vi "RHRT-IGVC-2013.vi"() -> ()   [LabVIEW 2011]
doc: "This the Rose-Hulman Robotics Tream IGVC compatition Code\nexample demonstrates the control of an autonomous robot through multiple asynchronous processes, modeled by VIs, that communicate with each other using shared variables. This example also shows an obstacle avoidance algorithm that the simulated robot uses as it navigates. The application includes the following processes:\n\n1. LIDAR Loop (\"Sense\")--Uses LabVIEW dataflow programming to generate simulated sensor data based on the position of the robot and any obstacles in the environment.\n\n2. Operator Loop (\"Think\")--Uses a state machine to control the movement of the robot according to commands from the user. When the robot follows a path without joystick or keyboard control, this process controls the attitude of the autonomous robot using a Vector Field Histogram (VFH) algorithm to avoid obstacles.\n\n3. Motor Loop (\"Act\")--Uses a Control and Simulation Loop, from the Control Design and Simulation Module, to create a model of the robot, simulate its dynamic behavior, and show the control loops and attitude observers."
uses:
  <vilib>/robotics/Controls/Compass Indicator/Compass Indicator.xctl
  <vilib>/Platform/TimedLoop/XDataNode/timing_clust.ctl
  <vilib>/Platform/TimedLoop/XDataNode/nitl_modes.ctl
  <vilib>/Platform/TimedLoop/XDataNode/wakeup.ctl
  <vilib>/Platform/TimedLoop/XDataNode/XDataNode.xnode
  <vilib>/Platform/TimedLoop/XDataNode/XDNodeRunTimeDep.lvlib
panel:
  out "Error":bool
  out "OK":bool
  in  "HUD 2":enum32{"GPS", "LIDAR", "IMU", "Occupancy Grid"}(tab)
  out "Health":u8(slide) scale=0.0..12.0
  out "XY Graph 2":cluster{dbl[], dbl[]}(graph)
  out "Data Aquired 2":picture
  out "Digree 2":dbl=16.3201904296875 caption="Digree"
  out "Compass Indicator 2":dbl(xcontrol)=16.3201904296875
  out "Occupancy Grid":dbl[][](graph)
  in  "Telemetry":T1(tab)
  out "Voltage":cluster{sgl, sgl, sgl}(knob)={13.4, 12.0, 47.48} caption="Main Battery Voltage\nInternal Voltage\nDSUB Voltage" scale=8.0..15.0
  out "Current":cluster{sgl, sgl, sgl, sgl}(knob)={0.0, 0.0, -2.0, -2.0} caption="Ch1 Motor Curret\nCh2 Motor Curret\nCh1 Battery Curret \nCh2 Battery Curret" scale=0.0..15.0
  out "IC Temp (C)":i32(slide)=22 scale=0.0..150.0
  out "Ch1 Temp (C)":i32(slide)=22 scale=0.0..150.0
  out "Ch2 Temp (C)":i32(slide)=23 scale=0.0..150.0
  out "Ch1 Encoder Speed\nCh2 Encoder Speed":cluster{i32, i32}(knob) scale=-300.0..300.0
  out "Image Out":T2(plugin-control)
  in  "Search For VISA":bool
  in  "HUD":T3(tab)=enum."Info"
  in  "Analog Stick":cluster{dbl, dbl}[](graph)
  in  "Clear Breadcrumbs":bool
  in  "Max Points":dbl=3000.0 format="%0.2f"
  out "XY Graph":cluster{dbl[], dbl[]}[](graph)
  out "Longitude Point":dbl format="%#_12g"
  out "Latitude Point":dbl format="%#_12g"
  out "Data Aquired":picture
  in  "Max Distance":dbl=3000.0 format="%0.2f"
  out "Digree":dbl=16.3201904296875
  out "Compass Indicator":dbl(xcontrol)=16.3201904296875
  out "Curretn POI":string
  in  "Curent Index":i32
  in  "Waypoint Table":string[][](table)=[["1.000000", "39.400000", "-87.200000"], ["2.000000", "39.600000", "-87.300000"], ["2.000000", "39.200000", "-87.400000"]]
  in  "Show GPS Diagram":bool
  in  "Show LL Diagram":bool
  in  "Show AI Diagram":bool
  in  "Show MCL Diagram":bool
  in  "About":bool
  in  "Stop":bool
  in  "Error Display":T4(tab)
  out "Cammera Status":bool
  out "Cammera Status 2":bool
  out "IMU Status":bool
  in  "IMU VISA":refnum<visa-resource-name>="COM7"
  out "Motor Status":bool
  in  "Motor VISA":refnum<visa-resource-name>="COM21"
  out "LIDAR Status":bool
  in  "LIDAR VISA":refnum<visa-resource-name>="COM20"
  out "GPS Status":bool
  in  "GPS VISA":refnum<visa-resource-name>="COM22"
  in  "GPS Error":errorcluster
  in  "LIDAR Error":errorcluster
  in  "Motor Error":errorcluster
  in  "IMU Error":errorcluster
  in  "Camera Error":errorcluster
  in  "Robot Mode:":T5(ring)
  out "End Loop":bool=TRUE
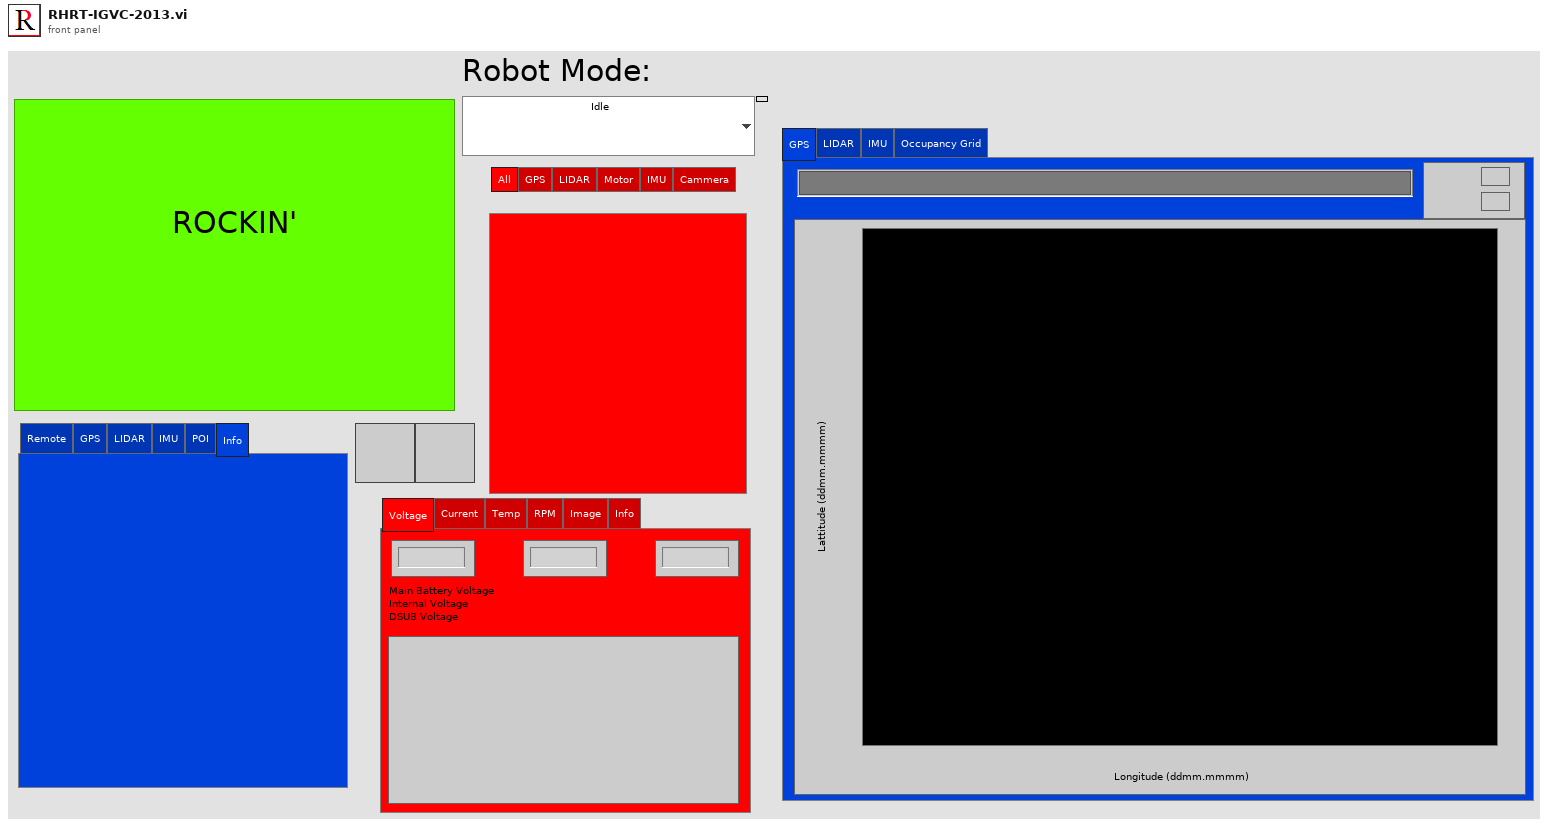
[diagram p1: front panel]
types:
  T1 = enum32{"Voltage", "Current", "Temp", "RPM", "Image", "Info"}
  T2 = typedef "IMAQ Image.ctl" = refnum<image>
  T3 = enum32{"Remote", "GPS", "LIDAR", "IMU", "POI", "Info"}
  T4 = enum32{"All", "GPS", "LIDAR", "Motor", "IMU", "Cammera"}
  T5 = enum16{"Idle", "Wiimote", "Joypad", "IGVC", "Avoide Objects", "Avoide Lines", "Path Planning", "Heading", "Waypoint"}
  T6 = typedef "XDNodeRunTimeDep.lvlib/timing_clust.ctl" = cluster{"Expected End [f-1]":u64, "Actual End [f-1]":u64, "Finished Late? [f-1]":bool, "Expected End [i-1]":u64, "Actual End [i-1]":u64, "Finished Late? [i-1]":bool, "Expected Start [i]":u64, "Actual Start [i]":u64, "Expected Start [f]":u64, "Actual Start [f]":u64, "Source Name":string, "Structure Name":string, "Period":i64, "Deadline":i64, "Offset":i64, "Start":i64, "Priority":i32, "Timeout":i32, "Mode":T7, "Wakeup Reason":T8, "Error":errorcluster, "Source Type":string, "Secondary Source Type":string, "Global End Time":u64, "Global Start Time":u64, "Frame Duration":u64, "Iteration Duration":u64, "Assigned CPU":i32, "I/O Scan Engine Mode":u32}
  T7 = typedef "XDNodeRunTimeDep.lvlib/nitl_modes.ctl" = enum32{"No Change", "Process missed periods, maintain original phase", "Discard missed periods, maintain original phase", "Process missed periods, ignore original phase", "Discard missed periods, ignore original phase"}
  T8 = typedef "XDNodeRunTimeDep.lvlib/wakeup.ctl" = enum32{"Normal", "Aborted", "Asynchronous wakeup", "Timing source error", "Timed loop error", "Timeout"}
  T9 = cluster{"Latitude":dbl, "Longitude":dbl, "Altitude":dbl, "Velocity, Correction & SET":cluster{"Velocity North":dbl, "Velocity East":dbl, "Velocity Up":dbl, "Ellipsoidal Height":dbl, "GDOP":sgl, "PDOP":sgl, "HDOP":sgl, "VDOP":sgl, "TDOP":sgl, "Horizontal Figure of Merit":u8, "Time Figure of Merit":u8, "Max dGPS Age":sgl, "Extended Navigation Mode":u8, "Antenna Height Adjustment ":dbl, "SET North":i32, "SET East":i32, "SET Up":i32}, "Time":cluster{"GPS Week":u16, "GPS Time of Week":sgl}, "Satellites Used":i32[]}
  T10 = cluster{"Azimuth":dbl, "FocusPointAltitude":dbl, "altMode":i32, "FocusPointLatitude":dbl, "FocusPointLongitude":dbl, "Range":dbl, "Tilt":dbl}
  T11 = cluster{"Position":cluster{"Roll":dbl, "Pitch":dbl, "Yaw":dbl}, "Orientation Matrix":dbl[][], "Magnetic Field":cluster{"Z-Axis Magnetic Field":dbl, "Y-Axis Magnetic Field":dbl, "X-Axis Magnetic Field":dbl}, "Acceleration":cluster{"Z-Axis Acceleration":dbl, "Y-Axis Acceleration":dbl, "X-Axis Acceleration":dbl}, "Angular Rate":cluster{"X-Axis Angular Rate":dbl, "Y-Axis Angular Rate":dbl, "Z-Axis Angular Rate":dbl}, "Quaternion":dbl[]}
  T12 = cluster{"Voltage":cluster{sgl, sgl, sgl}, "Encoder Speed":cluster{i32, i32}, "Temps":cluster{"IC Temp (C)":i32, "Ch1 Temp (C)":i32, "Ch2 Temp (C)":i32}, "Current":cluster{dbl, dbl, dbl, dbl}}
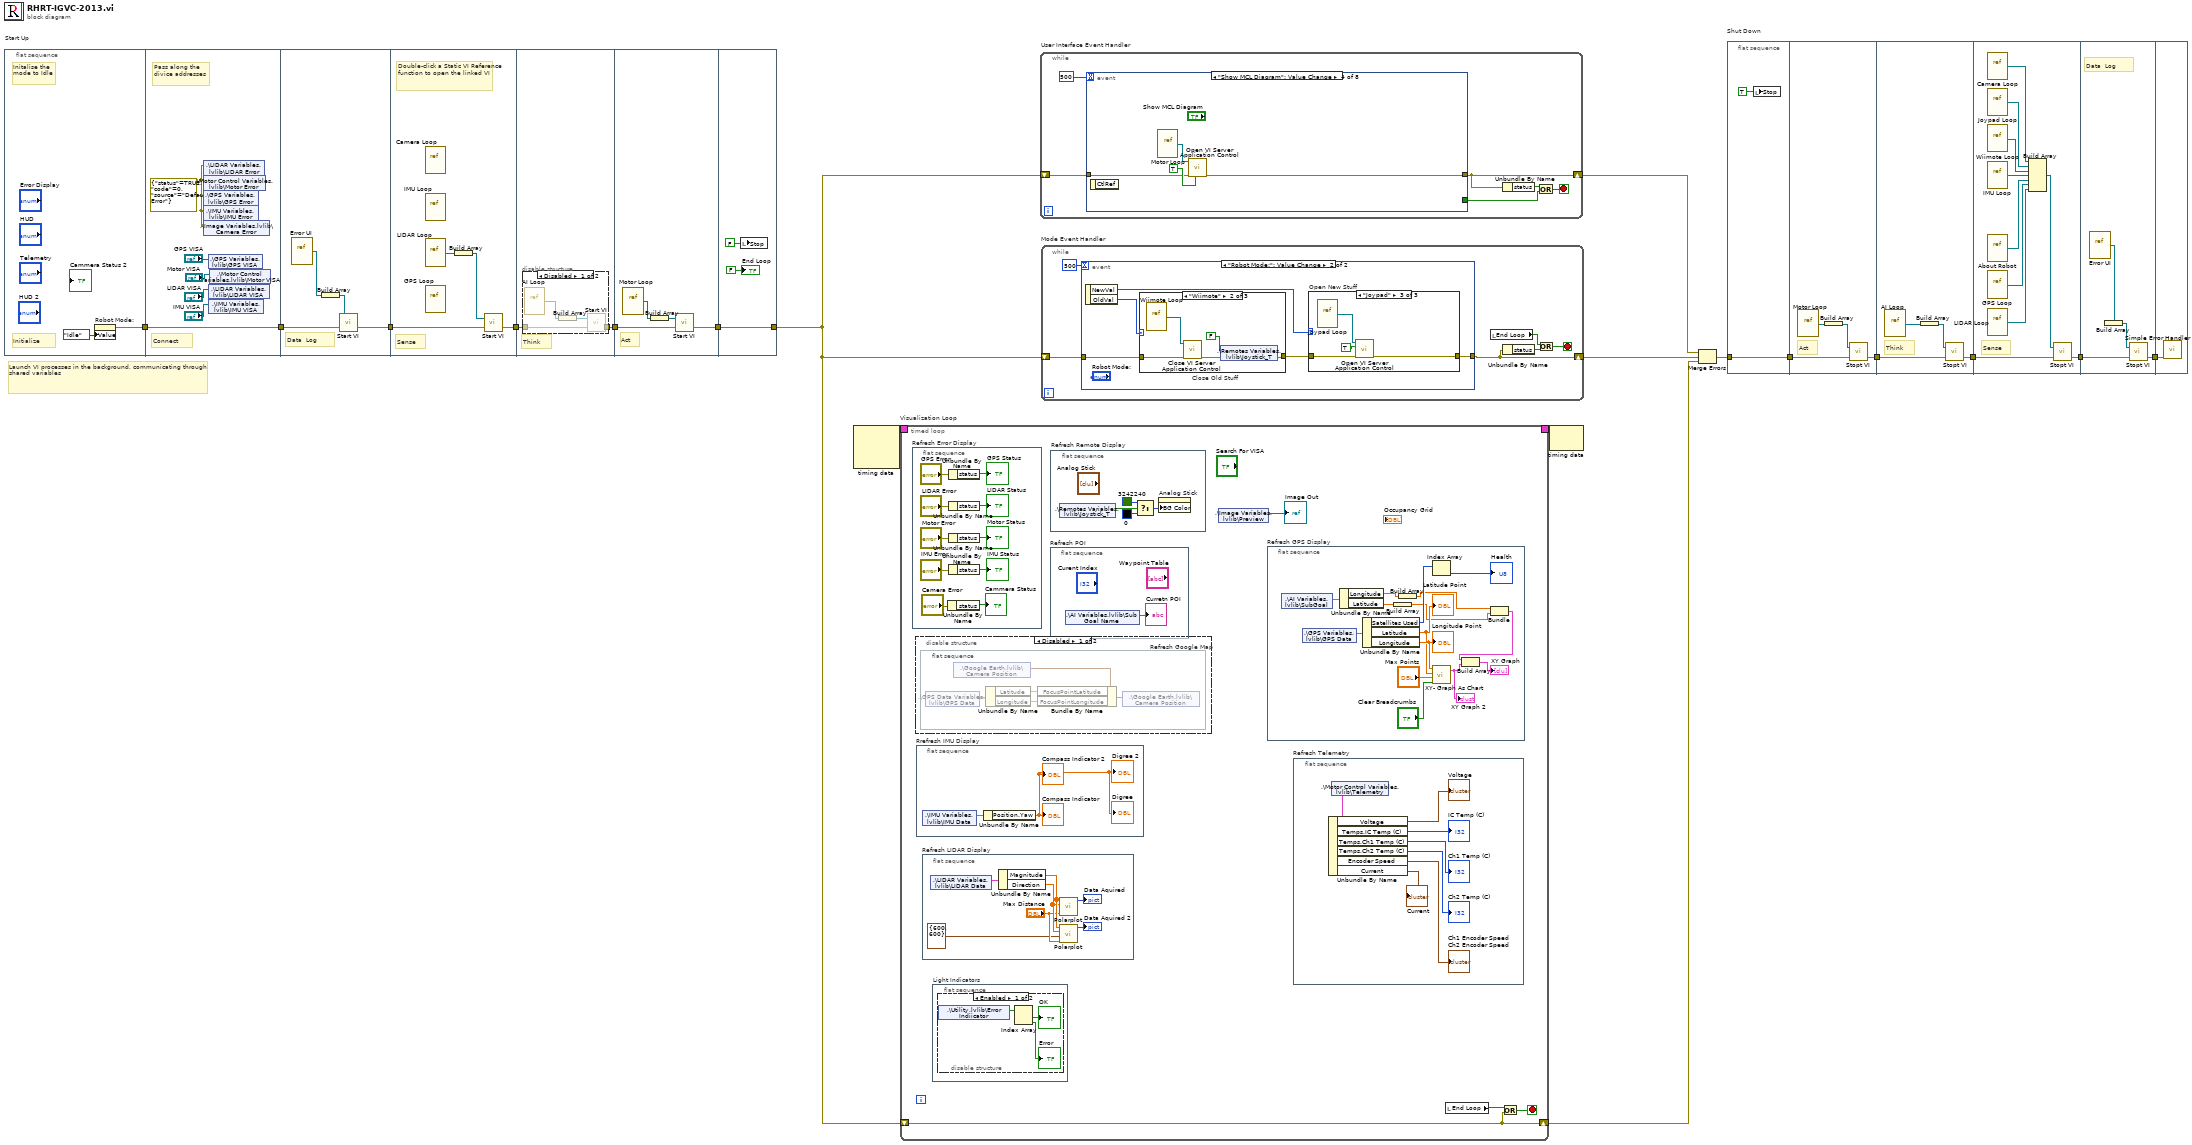
[diagram p0: block diagram]
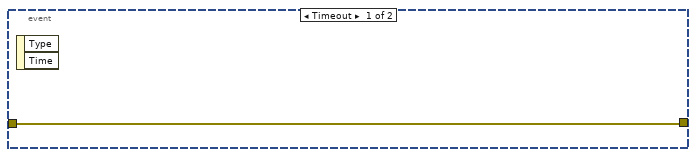
[diagram p2: hidden frame]
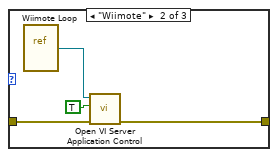
[diagram p4: hidden frame]
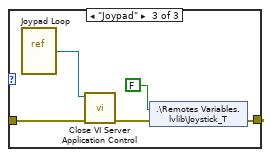
[diagram p6: hidden frame]
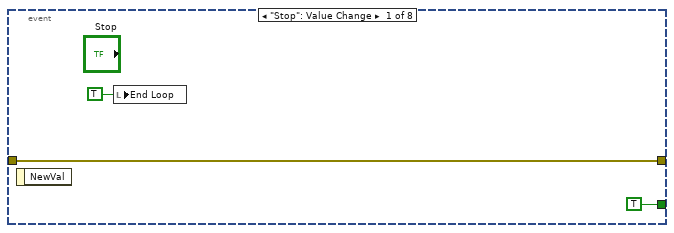
[diagram p8: hidden frame]
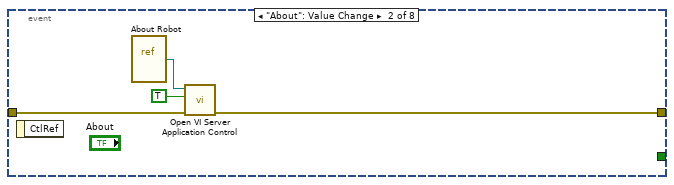
[diagram p9: hidden frame]
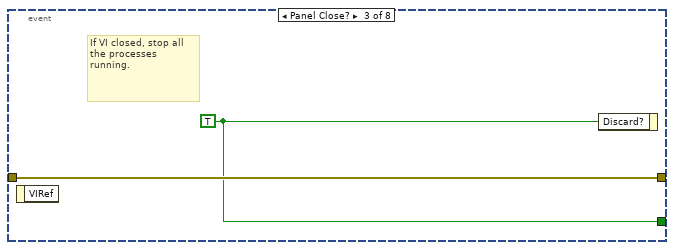
[diagram p10: hidden frame]
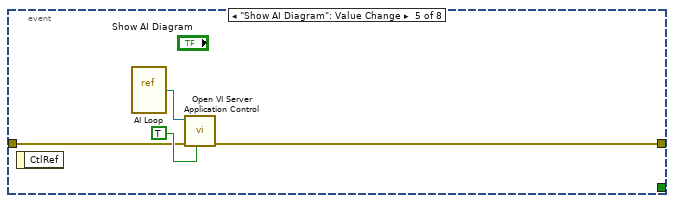
[diagram p11: hidden frame]
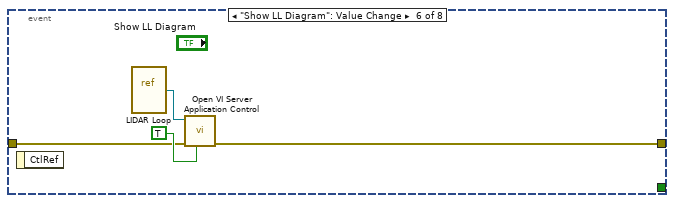
[diagram p12: hidden frame]
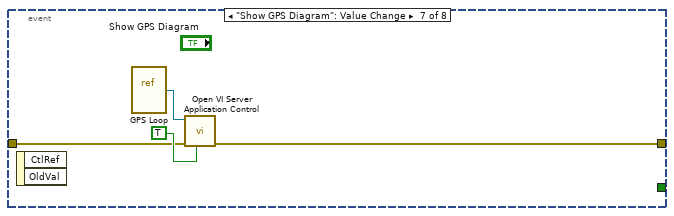
[diagram p13: hidden frame]
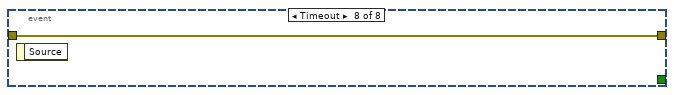
[diagram p14: hidden frame]
diagram:
  # "Launch VI processes in the background, communicating through shared variables"
  n1 = flat-sequence "Start Up" {
    tunnel: [w20] -> w13
    tunnel: [w23] -> w5
    tunnel: w13 -> [w23]
    tunnel: w5 -> [w30]
    tunnel: [w29] -> w1
    tunnel: [w32] -> w12
    tunnel: w1 -> [w33]
    tunnel: w12 -> [w36]
    tunnel: [w35] -> w10
    tunnel: [w44] -> w11
    tunnel: w10 -> [w45]
    tunnel: [w48] -> w6
    tunnel: w11 -> [w48]
    frame #0 {
      # "Initialize"
      # "Initalise the mode to Idle"
      n2 = property on="Robot Mode:" class="Enum (strict)"("Value"=T5."Idle" ("Robot Mode:")) -> (error out=w20:errorcluster)  [unwired: 2 in, 1 out]
    }
    frame #1 {
      w21 = errorcluster {"status"=TRUE, "code"=0, "source"="Default Error"} ("error out")
      # "Connect"
      # "Pass along the divice addresses"
      n3 = shared-variable ".\\LIDAR Variables.lvlib\\LIDAR Error"(w21) -> ()  [unwired: 1 in, 1 out]
      n4 = shared-variable ".\\Motor Control Variables.lvlib\\Motor Error"(w21) -> ()  [unwired: 1 in, 1 out]
      n5 = shared-variable ".\\GPS Variables.lvlib\\GPS Error"(w21) -> ()  [unwired: 1 in, 1 out]
      n6 = shared-variable ".\\IMU Variables.lvlib\\IMU Error"(w21) -> ()  [unwired: 1 in, 1 out]
      n7 = shared-variable ".\\Image Variables.lvlib\\Camera Error"(w21) -> ()  [unwired: 1 in, 1 out]
      n8 = shared-variable ".\\GPS Variables.lvlib\\GPS VISA"("GPS VISA") -> ()  [unwired: 1 in, 1 out]
      n9 = shared-variable ".\\LIDAR Variables.lvlib\\LIDAR VISA"("LIDAR VISA") -> ()  [unwired: 1 in, 1 out]
      n10 = shared-variable ".\\IMU Variables.lvlib\\IMU VISA"("IMU VISA") -> ()  [unwired: 1 in, 1 out]
      n11 = shared-variable ".\\Motor Control Variables.lvlib\\Motor VISA"("Motor VISA") -> ()  [unwired: 1 in, 1 out]
    }
    frame #2 {
      # "Data  Log"
      n12 = vi-ref "Error UI.vi"() -> (w27:refnum<vi>)
      n13 = Build Array(w27) -> (w28:refnum<vi>[])
      n14 = call "Start VI.vi"("error in"=w30, "VI refnum"=w28) -> ("error out"=w29:errorcluster)  [unwired: 1 in]
    }
    frame #3 {
      # "Double-click a Static VI Reference function to open the linked VI"
      # "Sense"
      n15 = vi-ref "Camera Loop.vi"() -> ()  [unwired: 1 out]
      n16 = vi-ref "IMU Loop.vi"() -> ()  [unwired: 1 out]
      n17 = vi-ref "LIDAR Loop.vi"() -> (w31:refnum<vi>)
      n18 = vi-ref "GPS Loop.vi"() -> ()  [unwired: 1 out]
      n19 = Build Array(w31) -> (w34:refnum<vi>[])
      n20 = call "Start VI.vi"("error in"=w33, "VI refnum"=w34) -> ("error out"=w32:errorcluster)  [unwired: 1 in]
    }
    frame #4 {
      # "Think"
      n21 = disable-structure shown="Disabled" {
        disable-tunnel: w36 -> [w40 w41]
        disable-tunnel: [w39 w41] -> w35
        frame Disabled {
          n22 = vi-ref "AI Loop.vi"() -> (w38:refnum<vi>)
          n23 = Build Array(w38) -> (w37:refnum<vi>[])
          n24 = call "Start VI.vi"("error in"=w40, "VI refnum"=w37) -> ("error out"=w39:errorcluster)  [unwired: 1 in]
        }
        frame Enabled {
        }
      }
    }
    frame #5 {
      # "Act"
      n25 = vi-ref "Motor Loop.vi"() -> (w43:refnum<vi>)
      n26 = Build Array(w43) -> (w42:refnum<vi>[])
      n27 = call "Start VI.vi"("error in"=w45, "VI refnum"=w42) -> ("error out"=w44:errorcluster)  [unwired: 1 in]
    }
    frame #6 {
      n28 = local write "Stop"(FALSE ("Halt TL")) -> ()
      "End Loop" <- FALSE ("Halt TL")
    }
  }
  n29 = node-c288() -> (w18:T6)  [unwired: 3 in]
  n30 = timed-loop "Visualization Loop" {
    timing: w18 -> [_]
    timing-out: [_] -> w17
    shift-right: [w49] -> w2
    shift-left: w6 -> [w49]
    stop <- w52 stop-if-true
    n31 = flat-sequence "Refresh Error Display" {
      frame #0 {
        n32 = Unbundle By Name("Camera Error") -> ("status"=→"Cammera Status":bool)
        n33 = Unbundle By Name("GPS Error") -> ("status"=→"GPS Status":bool)
        n34 = Unbundle By Name("LIDAR Error") -> ("status"=→"LIDAR Status":bool)
        n35 = Unbundle By Name("Motor Error") -> ("status"=→"Motor Status":bool)
        n36 = Unbundle By Name("IMU Error") -> ("status"=→"IMU Status":bool)
      }
    }
    n37 = disable-structure shown="Disabled" {
      frame Disabled {
        n38 = flat-sequence "Refresh Google Map" {
          frame #0 {
            n39 = shared-variable ".\\GPS Data Variables.lvlib\\GPS Data"() -> (w56:T9)  [unwired: 1 in, 1 out]
            n40 = shared-variable ".\\Google Earth.lvlib\\Camera Position"() -> (w57:T10)  [unwired: 1 in, 1 out]
            n41 = Unbundle By Name(w56) -> ("Latitude"=w53:dbl, "Longitude"=w55:dbl)
            n42 = Bundle By Name(cluster=w57, "FocusPointLatitude"=w53, "FocusPointLongitude"=w55) -> (w54:T10)
            n43 = shared-variable ".\\Google Earth.lvlib\\Camera Position"(w54) -> ()  [unwired: 1 in, 1 out]
          }
        }
      }
      frame Enabled {
      }
    }
    n44 = flat-sequence "Rrefresh IMU Display" {
      frame #0 {
        n45 = shared-variable ".\\IMU Variables.lvlib\\IMU Data"() -> (w85:T11)  [unwired: 1 in, 1 out]
        n46 = Unbundle By Name(w85) -> ("Position.Yaw"=→"Compass Indicator" →"Digree" →"Compass Indicator 2" →"Digree 2":dbl)
      }
    }
    n47 = flat-sequence "Refresh LIDAR Display" {
      frame #0 {
        n48 = shared-variable ".\\LIDAR Variables.lvlib\\LIDAR Data"() -> (w67:cluster{"Magnitude":dbl[], "Direction":dbl[]})  [unwired: 1 in, 1 out]
        n49 = Unbundle By Name(w67) -> ("Magnitude"=w64:dbl[], "Direction"=w63:dbl[])
        n50 = call "Polarplot.vi"("maximum"="Max Distance", "Direction"=w63, "Magnitude"=w64) -> ("Data Aquired"=→"Data Aquired":picture)  [unwired: 8 in]
        n51 = call "Polarplot.vi"("maximum"="Max Distance", "dimensions (w,h)"=cluster{"width":i16, "height":i16} {"width"=600, "height"=600}, "Direction"=w63, "Magnitude"=w64) -> ("Data Aquired"=→"Data Aquired 2":picture)  [unwired: 7 in]
      }
    }
    n52 = flat-sequence "Light Indicators" {
      frame #0 {
        n53 = disable-structure shown="Enabled" {
          frame Enabled {
            n54 = shared-variable ".\\Utility.lvlib\\Error Indiicator"() -> (w60:bool[])  [unwired: 1 in, 1 out]
            n55 = Index Array(array=w60) -> (element #1=→"OK":bool, element #2=→"Error":bool)  [unwired: 2 in]
          }
          frame Disabled {
          }
        }
      }
    }
    n56 = flat-sequence "Refresh POI" {
      frame #0 {
        n57 = shared-variable ".\\AI Variables.lvlib\\Sub Goal Name"() -> (→"Curretn POI":string)  [unwired: 1 in, 1 out]
      }
    }
    n58 = flat-sequence "Refresh Remote Display" {
      frame #0 {
        n59 = shared-variable ".\\Remotes Variables.lvlib\\Joystick_T"() -> (w94:bool)  [unwired: 1 in, 1 out]
        n60 = Select(t=u32 3242240, s=w94, f=u32 0) -> (s? t:f=w93:u32)
        n61 = property on="Analog Stick" class="XYGraph (strict)"("BG Color"=w93) -> ()  [unwired: 2 in, 2 out]
      }
    }
    n62 = shared-variable ".\\Image Variables.lvlib\\Preview"() -> (→"Image Out":refnum<image>)  [unwired: 1 in, 1 out]
    n63 = flat-sequence "Refresh GPS Display" {
      frame #0 {
        n64 = shared-variable ".\\AI Variables.lvlib\\SubGoal"() -> (w78:T9)  [unwired: 1 in, 1 out]
        n65 = shared-variable ".\\GPS Variables.lvlib\\GPS Data"() -> (w82:T9)  [unwired: 1 in, 1 out]
        n66 = Unbundle By Name(w78) -> ("Longitude"=w73:dbl, "Latitude"=w72:dbl)
        n67 = Unbundle By Name(w82) -> ("Satellites Used"=w79:i32[], "Latitude"=w76:dbl, "Longitude"=w77:dbl)
        "Latitude Point" <- w76
        "Longitude Point" <- w77
        n68 = Build Array(w72) -> (w70:dbl[])
        n69 = Build Array(w73) -> (w71:dbl[])
        n70 = Index Array(array=w79) -> (element=→"Health":i32)  [unwired: 1 in]
        n71 = call "XY- Graph As Chart.vi"("Clear Graph (F)"="Clear Breadcrumbs", "Maxi Points (10,000)"="Max Points", "Y-Value"=w76, "X- Value"=w77) -> ("XY Graph"=w75:cluster{dbl[], dbl[]})  [unwired: 1 out]
        "XY Graph 2" <- w75
        n72 = Bundle(w71, w70) -> (w69:cluster{dbl[], dbl[]})  [unwired: 1 out]
        n73 = Build Array(w69, w75) -> (→"XY Graph":cluster{dbl[], dbl[]}[])
      }
    }
    n74 = flat-sequence "Refresh Telemetry" {
      frame #0 {
        n75 = shared-variable ".\\Motor Control Variables.lvlib\\Telemetry"() -> (w92:T12)  [unwired: 1 in, 1 out]
        n76 = Unbundle By Name(w92) -> ("Voltage"=→"Voltage":cluster{sgl, sgl, sgl}, "Temps.IC Temp (C)"=→"IC Temp (C)":i32, "Temps.Ch1 Temp (C)"=→"Ch1 Temp (C)":i32, "Temps.Ch2 Temp (C)"=→"Ch2 Temp (C)":i32, "Encoder Speed"=→"Ch1 Encoder Speed\nCh2 Encoder Speed":cluster{i32, i32}, "Current"=→"Current":cluster{dbl, dbl, dbl, dbl})
      }
    }
    n77 = local read "End Loop"() -> (w50:bool)
    n78 = Or(x=w50, y=w49) -> (x .or. y?=w52:bool)
  }
  n79 = while "User Interface Event Handler" {
    shift-right: [w111] -> w16
    shift-left: w6 -> [w114]
    stop <- w113 stop-if-true
    n80 = event shown="[3] \"Show MCL Diagram\": Value Change" {
      selector: _ -> [_ _ _ _ _ _ _ _]
      dyn-events: _ -> [_ _ _ _ _ _ _ _]
      timeout: 500 -> [_ _ _ _ _ _ _ _]
      tunnel: [TRUE _ w122 _ _ _ _ _] -> w109
      tunnel: w114 -> [w117 w120 w123 w125 w129 w133 w136 w140]
      tunnel: [w117 w119 w123 w124 w128 w132 w137 w140] -> w111
      event "Stop": Value Change {
        n81 = event-data() -> ()  [unwired: 2 out]
        n82 = local write "End Loop"(TRUE ("End Loop")) -> ()
      }
      event "About": Value Change {
        n83 = event-data() -> ()  [unwired: 2 out]
        n84 = vi-ref "About Robot.vi"() -> (w121:refnum<vi>)
        n85 = call "Open VI Server Application Control.vi"("error in (no error)"=w120, "run VI (F)"=TRUE ("Launch Map"), "VI refnum"=w121) -> ("error out"=w119:errorcluster)  [unwired: 8 in]
      }
      event Panel Close? {
        w122 = TRUE ("Discard?")
        # "If VI closed, stop all the processes running."
        n86 = event-data() -> ()  [unwired: 2 out]
        n87 = event-data("Discard?"=w122) -> ()  [unwired: 1 in, 1 out]
      }
      event "Show MCL Diagram": Value Change {
        n88 = event-data() -> ()  [unwired: 2 out]
        n89 = vi-ref "Motor Loop.vi"() -> (w127:refnum<vi>)
        n90 = call "Open VI Server Application Control.vi"("open block diagram (F)"=TRUE ("Open Front Panel"), "error in (no error)"=w125, "VI refnum"=w127) -> ("error out"=w124:errorcluster)  [unwired: 8 in]
      }
      event "Show AI Diagram": Value Change {
        n91 = event-data() -> ()  [unwired: 2 out]
        n92 = vi-ref "AI Loop.vi"() -> (w130:refnum<vi>)
        n93 = call "Open VI Server Application Control.vi"("open block diagram (F)"=TRUE ("Open Front Panel"), "error in (no error)"=w129, "VI refnum"=w130) -> ("error out"=w128:errorcluster)  [unwired: 8 in]
      }
      event "Show LL Diagram": Value Change {
        n94 = event-data() -> ()  [unwired: 2 out]
        n95 = vi-ref "LIDAR Loop.vi"() -> (w134:refnum<vi>)
        n96 = call "Open VI Server Application Control.vi"("open block diagram (F)"=TRUE ("Open Front Panel"), "error in (no error)"=w133, "VI refnum"=w134) -> ("error out"=w132:errorcluster)  [unwired: 8 in]
      }
      event "Show GPS Diagram": Value Change {
        n97 = event-data() -> ()  [unwired: 3 out]
        n98 = vi-ref "GPS Loop.vi"() -> (w138:refnum<vi>)
        n99 = call "Open VI Server Application Control.vi"("open block diagram (F)"=TRUE ("Open Front Panel"), "error in (no error)"=w136, "VI refnum"=w138) -> ("error out"=w137:errorcluster)  [unwired: 8 in]
      }
      event Timeout {
        n100 = event-data() -> ()  [unwired: 2 out]
      }
    }
    n101 = Unbundle By Name(w111) -> ("status"=w110:bool)
    n102 = Or(x=w110, y=w109) -> (x .or. y?=w113:bool)
  }
  n103 = while "Mode Event Handler" {
    shift-right: [w143] -> w7
    shift-left: w6 -> [w144]
    stop <- w145 stop-if-true
    n104 = event shown="[1] \"Robot Mode:\": Value Change" {
      selector: _ -> [_ _]
      dyn-events: _ -> [_ _]
      timeout: 500 -> [_ _]
      tunnel: [w147 w150] -> w143
      tunnel: w144 -> [w147 w152]
      event Timeout {
        n105 = event-data() -> ()  [unwired: 1 in, 2 out]
      }
      event "Robot Mode:": Value Change {
        n106 = event-data() -> ("NewVal"=w149:T5, "OldVal"=w148:T5)  [unwired: 1 in]
        n107 = case "Close Old Stuff" shown="\"Wiimote\"" w148 {
          tunnel: w152 -> [w162 w167 w172]
          tunnel: [w162 w163 w168] -> w151
          frame "Idle", Default {
          }
          frame "Wiimote" {
            n108 = vi-ref "Wiimote Loop.vi"() -> (w166:refnum<vi>)
            n109 = call "Close VI Server Application Control.vi"("error in (no error)"=w167, "VI refnum"=w166) -> ("error out"=w164:errorcluster)  [unwired: 9 in]
            n110 = shared-variable ".\\Remotes Variables.lvlib\\Joystick_T"(FALSE ("Joystick_T"), error in=w164) -> (error out=w163:errorcluster)
          }
          frame "Joypad" {
            n111 = vi-ref "Joypad Loop.vi"() -> (w171:refnum<vi>)
            n112 = call "Close VI Server Application Control.vi"("error in (no error)"=w172, "VI refnum"=w171) -> ("error out"=w169:errorcluster)  [unwired: 9 in]
            n113 = shared-variable ".\\Remotes Variables.lvlib\\Joystick_T"(FALSE ("Joystick_T"), error in=w169) -> (error out=w168:errorcluster)
          }
        }
        n114 = case "Open New Stuff" shown="\"Joypad\"" w149 {
          tunnel: w151 -> [w153 w157 w161]
          tunnel: [w153 w155 w159] -> w150
          frame "Idle", Default {
          }
          frame "Wiimote" {
            n115 = vi-ref "Wiimote Loop.vi"() -> (w154:refnum<vi>)
            n116 = call "Open VI Server Application Control.vi"("error in (no error)"=w157, "run VI (F)"=TRUE, "VI refnum"=w154) -> ("error out"=w155:errorcluster)  [unwired: 8 in]
          }
          frame "Joypad" {
            n117 = vi-ref "Joypad Loop.vi"() -> (w158:refnum<vi>)
            n118 = call "Open VI Server Application Control.vi"("error in (no error)"=w161, "run VI (F)"=TRUE, "VI refnum"=w158) -> ("error out"=w159:errorcluster)  [unwired: 8 in]
          }
        }
      }
    }
    n119 = local read "End Loop"() -> (w142:bool)
    n120 = Unbundle By Name(w143) -> ("status"=w146:bool)
    n121 = Or(x=w142, y=w146) -> (x .or. y?=w145:bool)
  }
  n122 = node-c288(w17) -> ()  [unwired: 1 out]
  n123 = Merge Errors(w16, w7, w2) -> (w14:errorcluster)
  n124 = flat-sequence "Shut Down" {
    tunnel: w14 -> [w173]
    tunnel: [w173] -> w15
    tunnel: w15 -> [w178]
    tunnel: [w177] -> w9
    tunnel: w9 -> [w182]
    tunnel: [w181] -> w8
    tunnel: w8 -> [w192]
    tunnel: [w191] -> w4
    tunnel: w4 -> [w194]
    tunnel: [w196] -> w3
    tunnel: w3 -> [w197]
    frame #0 {
      n125 = local write "Stop"(TRUE ("Halt TL")) -> ()
    }
    frame #1 {
      # "Act"
      n126 = vi-ref "Motor Loop.vi"() -> (w176:refnum<vi>)
      n127 = Build Array(w176) -> (w175:refnum<vi>[])
      n128 = call "Stopt VI.vi"("error in"=w178, "VI refnum"=w175) -> ("error out"=w177:errorcluster)  [unwired: 1 in]
    }
    frame #2 {
      # "Think"
      n129 = vi-ref "AI Loop.vi"() -> (w179:refnum<vi>)
      n130 = Build Array(w179) -> (w180:refnum<vi>[])
      n131 = call "Stopt VI.vi"("error in"=w182, "VI refnum"=w180) -> ("error out"=w181:errorcluster)  [unwired: 1 in]
    }
    frame #3 {
      # "Sense"
      n132 = vi-ref "Camera Loop.vi"() -> (w183:refnum<vi>)
      n133 = vi-ref "Joypad Loop.vi"() -> (w184:refnum<vi>)
      n134 = vi-ref "Wiimote Loop.vi"() -> (w185:refnum<vi>)
      n135 = vi-ref "IMU Loop.vi"() -> (w186:refnum<vi>)
      n136 = vi-ref "About Robot.vi"() -> (w189:refnum<vi>)
      n137 = vi-ref "GPS Loop.vi"() -> (w188:refnum<vi>)
      n138 = vi-ref "LIDAR Loop.vi"() -> (w187:refnum<vi>)
      n139 = Build Array(w183, w184, w185, w186, w189, w188, w187) -> (w190:refnum<vi>[])
      n140 = call "Stopt VI.vi"("error in"=w192, "VI refnum"=w190) -> ("error out"=w191:errorcluster)  [unwired: 1 in]
    }
    frame #4 {
      # "Data  Log"
      n141 = vi-ref "Error UI.vi"() -> (w193:refnum<vi>)
      n142 = Build Array(w193) -> (w195:refnum<vi>[])
      n143 = call "Stopt VI.vi"("error in"=w194, "VI refnum"=w195) -> ("error out"=w196:errorcluster)  [unwired: 1 in]
    }
    frame #5 {
      n144 = call <vilib>:"Simple Error Handler.vi"("error in (no error)"=w197) -> ()  [unwired: 4 in, 5 out]
    }
  }
